vi "Write.vi"(8 "error in (no error)":errorcluster, 10 "Array":string[][](array[string]), 11 "Saving OO in":refnum<class "Saving OO.lvclass">) -> (0 "error out":errorcluster, 3 "Saving OO out":refnum<class "Saving OO.lvclass">)   [LabVIEW 2020, in "Saving OO.lvclass"]
uses:
  Saving OO.lvclass
  Saving OO.lvclass/Saving OO.ctl
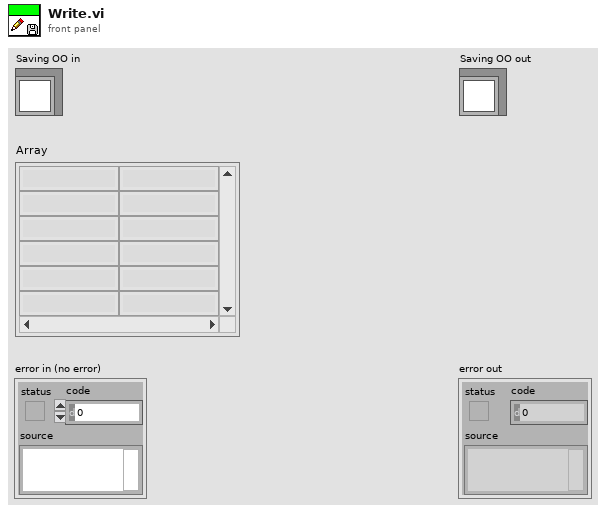
[diagram p1: front panel]
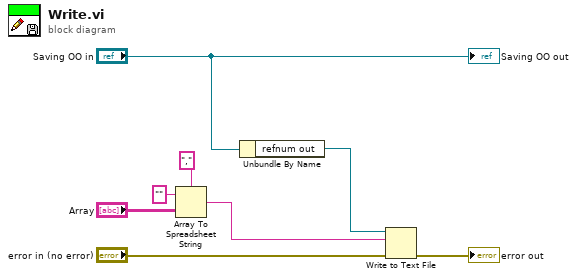
[diagram p0: block diagram]
diagram:
  n1 = Array To Spreadsheet String(delimiter (Tab)=",", array="Array", 3:"" ("format string")) -> (spreadsheet string=w6:string)
  n2 = Unbundle By Name("Saving OO in") -> ("refnum out"=w1:refnum<file>)
  n3 = Write to Text File(file (use dialog)=w1, text=w6, error in="error in (no error)") -> (error out=→"error out":errorcluster)  [unwired: 1 in, 2 out]
  "Saving OO out" <- "Saving OO in"
